vi "Initialize Queues.vi"(8 "error in (no error)":errorcluster) -> (0 "error out":errorcluster, 3 "output cluster":T1)   [LabVIEW 2024]
uses:
  Message Queues.ctl
  Message Cluster.ctl
  Message.ctl
  Washing Control Cluster.ctl
  States of Washing.ctl
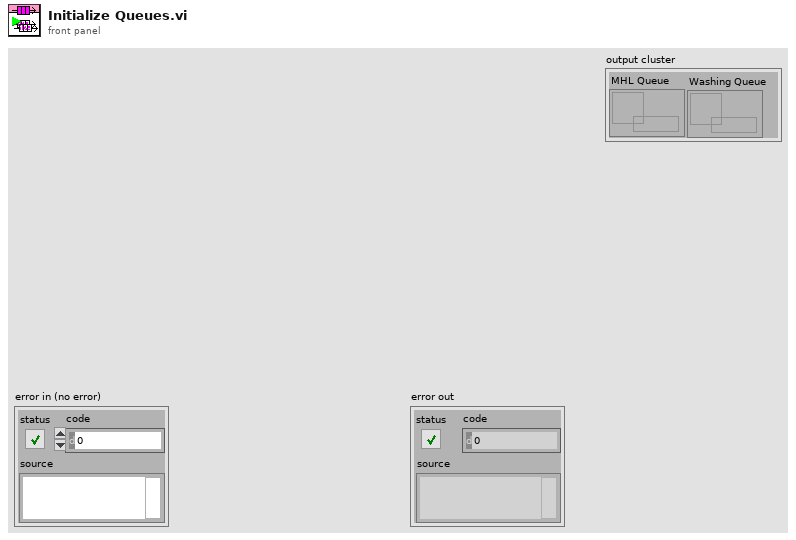
[diagram p1: front panel]
types:
  T1 = typedef "Message Queues.ctl" = cluster{"MHL Queue":refnum<queue>, "Washing Queue ":refnum<queue>}
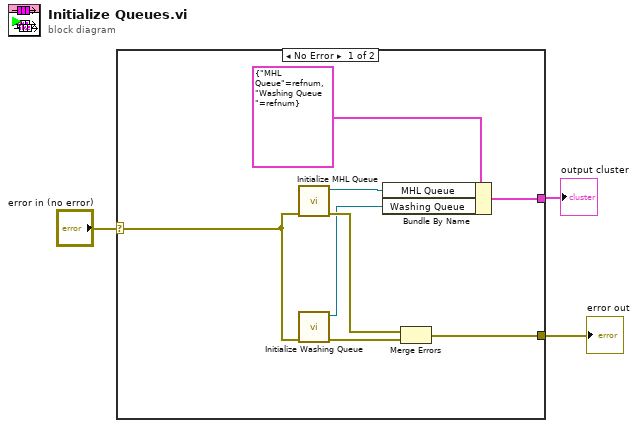
[diagram p0: block diagram]
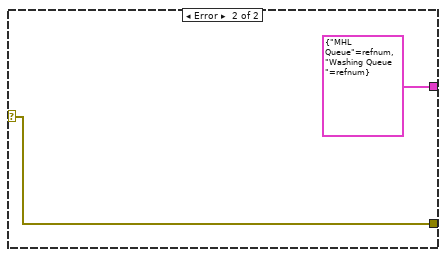
[diagram p2: hidden frame]
diagram:
  n1 = case shown="No Error" "error in (no error)" {
    selector: "error in (no error)" -> [w5 w13]
    tunnel: [w9 T1 {"MHL Queue"=refnum, "Washing Queue "=refnum} ("Message Queues")] -> w3
    tunnel: [w6 w13] -> w2
    frame No Error {
      n2 = call "Initialize MHL Queue.vi"("error in (no error)"=w5) -> ("Queue out"=w10:refnum<queue>, "error out"=w8:errorcluster)  [unwired: 8 in]
      n3 = call "Initialize Washing Queue.vi"("error in (no error)"=w5) -> ("queue out"=w4:refnum<queue>, "error out"=w7:errorcluster)  [unwired: 8 in]
      n4 = Bundle By Name(cluster=T1 {"MHL Queue"=refnum, "Washing Queue "=refnum} ("Message Queues"), "MHL Queue"=w10, "Washing Queue"=w4) -> (w9:T1)
      n5 = Merge Errors(w8, w7) -> (w6:errorcluster)
    }
    frame Error {
    }
  }
  "error out" <- w2
  "output cluster" <- w3
